vi "conversion 2.vi"(8 "Channel Indices":u8[](array[numeric]), 11 "voltage data":sgl[](array[numeric]) format="%.5f") -> (1 "Out of Range":bool[](array[boolean]), 3 "calibrated data":sgl[](array[numeric]) format="%.5f")   [LabVIEW 2012]
uses:
  global scale array.vi
  DataServer/Server Stats.vi
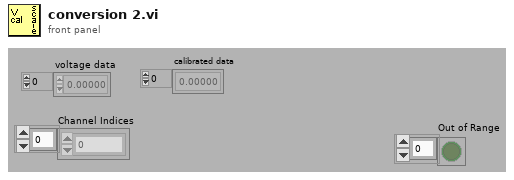
[diagram p1: front panel]
types:
  T1 = typedef "calib array.ctl" = T2[]
  T2 = typedef "conversion.ctl" = cluster{"conversion matrix":sgl[][], "units":string, "name":string, "scale type":T3, "offset (volts)":dbl, "second channel":i8, "correspondence table":T4, "offset (physical units)":dbl, "pH scale":T5, "D.O.":T6}
  T3 = typedef "scale type.ctl" = enum16{"Volts", "Polynomial", "Correspondence Table", "pH", "Dissolved Oxygen", "Quadratic"}
  T4 = typedef "correspondence table.ctl" = cluster{"physical units":dbl, "volts":dbl}[]
  T5 = typedef "pH scale.ctl" = cluster{"Buffers":cluster{"Buffer":dbl, "Calibrated":bool, "V/T":dbl}[], "Temperature":dbl}
  T6 = typedef "DO scale.ctl" = cluster{"Temperature":dbl, "K":dbl, "barometric pressure":dbl}
  T7 = typedef "Server stats.ctl" = cluster{"scan rate":dbl, "# connections":i32, "channel settings":cluster{"Name":string, "upper input limits":sgl, "lower input limits":sgl, "Location":string}[]}
  T8 = cluster{"Name":string, "upper input limits":sgl, "lower input limits":sgl, "Location":string}[]
  T9 = cluster{"Name":string, "upper input limits":sgl, "lower input limits":sgl, "Location":string}
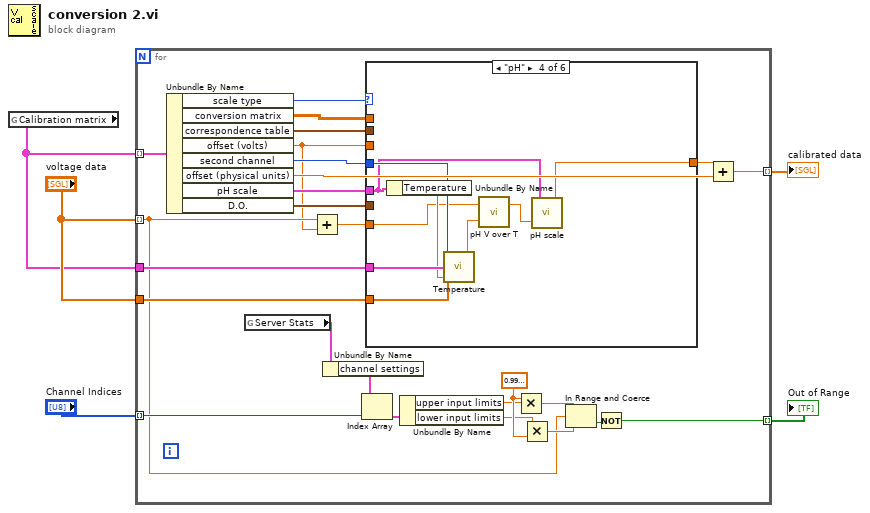
[diagram p0: block diagram]
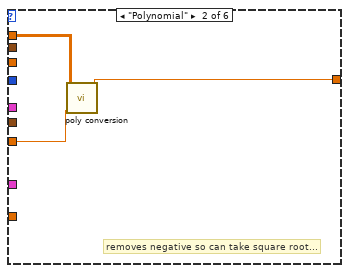
[diagram p3: hidden frame]
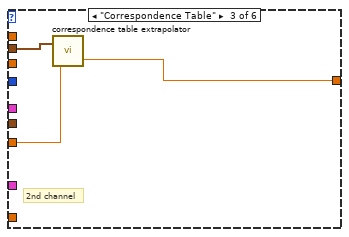
[diagram p4: hidden frame]
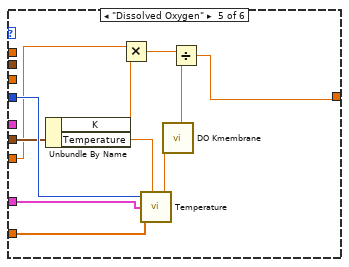
[diagram p5: hidden frame]
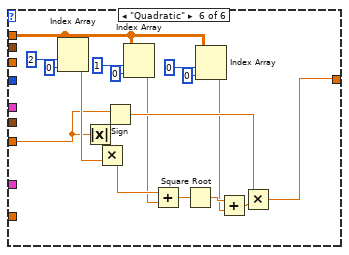
[diagram p6: hidden frame]
diagram:
  n1 = global read "global scale array.vi" "Calibration matrix"() -> (w1:T1)
  n2 = for {
    tunnel: w1 -> [w10] mode=indexing
    tunnel: "voltage data" -> [w8] mode=indexing
    tunnel: "voltage data" -> [w25]
    tunnel: [w24] -> w4 mode=indexing
    tunnel: [w16] -> w3 mode=indexing
    tunnel: "Channel Indices" -> [w15] mode=indexing
    tunnel: w1 -> [w11]
    w23 = sgl 0.99 ("x")
    n3 = Unbundle By Name(w10) -> ("scale type"=w30:T3, "conversion matrix"=w31:sgl[][], "correspondence table"=w29:T4, "offset (volts)"=w7:dbl, "second channel"=w26:i8, "offset (physical units)"=w27:dbl, "pH scale"=w13:T5, "D.O."=w12:T6)
    n4 = global read "Server Stats.vi" "Server Stats"() -> (w9:T7)
    n5 = Add(x=w8, y=w7) -> (x+y=w6:dbl)
    n6 = Unbundle By Name(w9) -> ("channel settings"=w17:T8)
    n7 = Index Array(array=w17, index=w15) -> (element=w14:T9)
    n8 = case shown="\"pH\"" w30 {
      tunnel: w31 -> [_ w35 _ _ _ w62]
      tunnel: [w32 w34 w37 w41 w58 w60] -> w28
      tunnel: w29 -> [_ _ w38 _ _ _]
      tunnel: w7 -> [_ _ _ _ _ _]
      tunnel: w26 -> [_ _ _ w47 w54 _]
      tunnel: w11 -> [_ _ _ w46 w56 _]
      tunnel: w25 -> [_ _ _ w45 w55 _]
      tunnel: w13 -> [_ _ _ w42 _ _]
      tunnel: w12 -> [_ _ _ _ w52 _]
      tunnel: w6 -> [w32 w33 w36 w39 w48 w59]
      frame "Volts", Default {
      }
      frame "Polynomial" {
        # "removes negative so can take square root..."
        n9 = call "poly conversion.vi"("Volts"=w33, "conversion matrix"=w35) -> ("Calibrated value"=w34:dbl)  [unwired: 9 in]
      }
      frame "Correspondence Table" {
        # "2nd channel"
        n10 = call "correspondence table extrapolator.vi"("Volts"=w36, "correspondence table"=w38) -> ("scaled"=w37:dbl)  [unwired: 1 out]
      }
      frame "pH" {
        n11 = Unbundle By Name(w42) -> ("Temperature"=w43:dbl)
        n12 = call "Temperature.vi"("second channel"=w47, "selected calibration array"=w46, "voltage data"=w45, "Default Temperature (C)"=w43) -> ("Temperature (C)"=w44:dbl)  [unwired: 1 in]
        n13 = call "pH V over T.vi"("Temperature"=w44, "Voltage"=w39) -> ("V/T"=w40:dbl)  [unwired: 1 out]
        n14 = call "pH scale.vi"("V/T"=w40, "pH scale"=w42) -> ("pH"=w41:dbl)  [unwired: 1 out]
      }
      frame "Dissolved Oxygen" {
        n15 = Unbundle By Name(w52) -> ("K"=w50:dbl, "Temperature"=w51:dbl)
        n16 = Multiply(x=w48, y=w50) -> (x*y=w49:dbl)
        n17 = call "Temperature.vi"("second channel"=w54, "selected calibration array"=w56, "voltage data"=w55, "Default Temperature (C)"=w51) -> ("Temperature (C)"=w53:dbl)  [unwired: 1 in]
        n18 = call "DO Kmembrane.vi"("Temperature (C)"=w53) -> ("Kmembrane"=w57:dbl)  [unwired: 10 in]
        n19 = Divide(x=w49, y=w57) -> (x/y=w58:dbl)
      }
      frame "Quadratic" {
        n20 = Index Array(array=w62, index (row)=2 ("Index"), index (col)=0 ("Disabled Index (col)")) -> (element=w68:sgl)
        n21 = Absolute Value(x=w59) -> (abs(x)=w72:dbl)
        n22 = Multiply(x=w72, y=w68) -> (x*y=w74:dbl)
        n23 = Sign(1:w59) -> (0:w69:dbl)
        n24 = Index Array(array=w62, index (row)=1 ("Index"), index (col)=0 ("Disabled Index (col)")) -> (element=w65:sgl)
        n25 = Add(x=w74, y=w65) -> (x+y=w73:dbl)
        n26 = Square Root(x=w73) -> (sqrt(x)=w71:dbl)
        n27 = Index Array(array=w62, index (row)=0 ("Index"), index (col)=0 ("Disabled Index (col)")) -> (element=w61:sgl)
        n28 = Add(x=w71, y=w61) -> (x+y=w70:dbl)
        n29 = Multiply(x=w69, y=w70) -> (x*y=w60:dbl)
      }
    }
    n30 = Unbundle By Name(w14) -> ("upper input limits"=w19:sgl, "lower input limits"=w20:sgl)
    n31 = Multiply(x=w23, y=w19) -> (x*y=w22:sgl)
    n32 = Multiply(x=w20, y=w23) -> (x*y=w21:sgl)
    n33 = In Range and Coerce(upper limit=w22, x=w8, lower limit=w21) -> (In Range?=w18:bool)  [unwired: 1 out]
    n34 = Not(x=w18) -> (.not. x?=w16:bool)
    n35 = Add(x=w28, y=w27) -> (x+y=w24:dbl)
  }
  "calibrated data" <- w4
  "Out of Range" <- w3
